vi "library_move.vi"(6 "lvlib_move_directory":path, 8 "error in (no error)":errorcluster, 11 "build_specifications":T1) -> (0 "error out":errorcluster)   [LabVIEW 2015, in "lv-builder-default.lvlib"]
uses:
  lv-builder-default.lvlib
  lv-build/public/_controls/build_specification.ctl
  lv-build/public/_controls/build_type.ctl
  lv-build/lv-build.lvlib
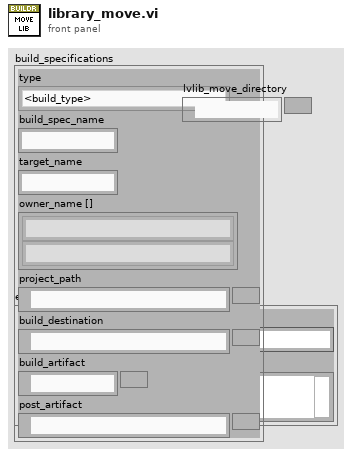
[diagram p1: front panel]
types:
  T1 = typedef "lv-build.lvlib/build_specification.ctl" = cluster{"type":T2, "build_spec_name":string, "target_name":string, "owner_name []":string[], "project_path":path, "build_destination":path, "build_artifact":path, "post_artifact":path}
  T2 = typedef "lv-build.lvlib/build_type.ctl" = enum16{"<build_type>", "application_pc", "application_rt", "installer", "llb", "lvlibp", "zip", "fpga", "<null>"}
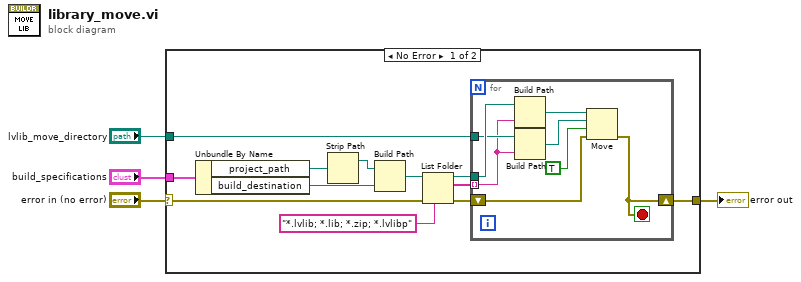
[diagram p0: block diagram]
diagram:
  n1 = case shown="No Error" "error in (no error)" {
    selector: "error in (no error)" -> [w13 w25]
    tunnel: [w6 w25] -> w4
    tunnel: "build_specifications" -> [w16 _]
    tunnel: "lvlib_move_directory" -> [w5 _]
    frame No Error {
      n2 = Unbundle By Name(w16) -> ("project_path"=w8:path, "build_destination"=w15:path)
      n3 = Strip Path(path=w8) -> (stripped path=w7:path)  [unwired: 1 out]
      n4 = Build Path(base path=w7, name or relative path=w15) -> (appended path=w14:path)
      n5 = List Folder(path=w14, pattern="*.lvlib; *.lib; *.zip; *.lvlibp", error in=w13) -> (path out=w9:path, filenames=w10:string[], error out=w12:errorcluster)  [unwired: 1 in, 1 out]
      n6 = for {
        tunnel: w10 -> [w19] mode=indexing
        shift-right: [w24] -> w6
        shift-left: w12 -> [w17]
        tunnel: w5 -> [w20]
        tunnel: w9 -> [w23]
        stop <- w24 stop-if-true
        n7 = Build Path(base path=w23, name or relative path=w19) -> (appended path=w22:path)
        n8 = Build Path(base path=w20, name or relative path=w19) -> (appended path=w18:path)
        n9 = Move(source path=w22, error in=w17, 9:TRUE ("overwrite (F)"), 10:w18) -> (error out=w24:errorcluster)  [unwired: 1 in, 2 out]
      }
    }
    frame Error {
    }
  }
  "error out" <- w4
